vi "OE2012&OE2022_USB_Query Data.vi"(0 "VISA resource name":refnum<visa-resource-name>, 11 "Error in (no error)":errorcluster caption="error out（no error）") -> (3 "Buffer Count":u8, 4 "VISA resource  out":refnum<visa-resource-name>, 6 "Parameter Values":T1, 8 "Total Date Array":dbl[][](array[numeric]), 10 "Output String":string, 13 "Trig_Count":u8[](array[numeric]), 14 "PLL&Overload":T2, 15 "Error out":errorcluster caption="error out")   [LabVIEW 2011]
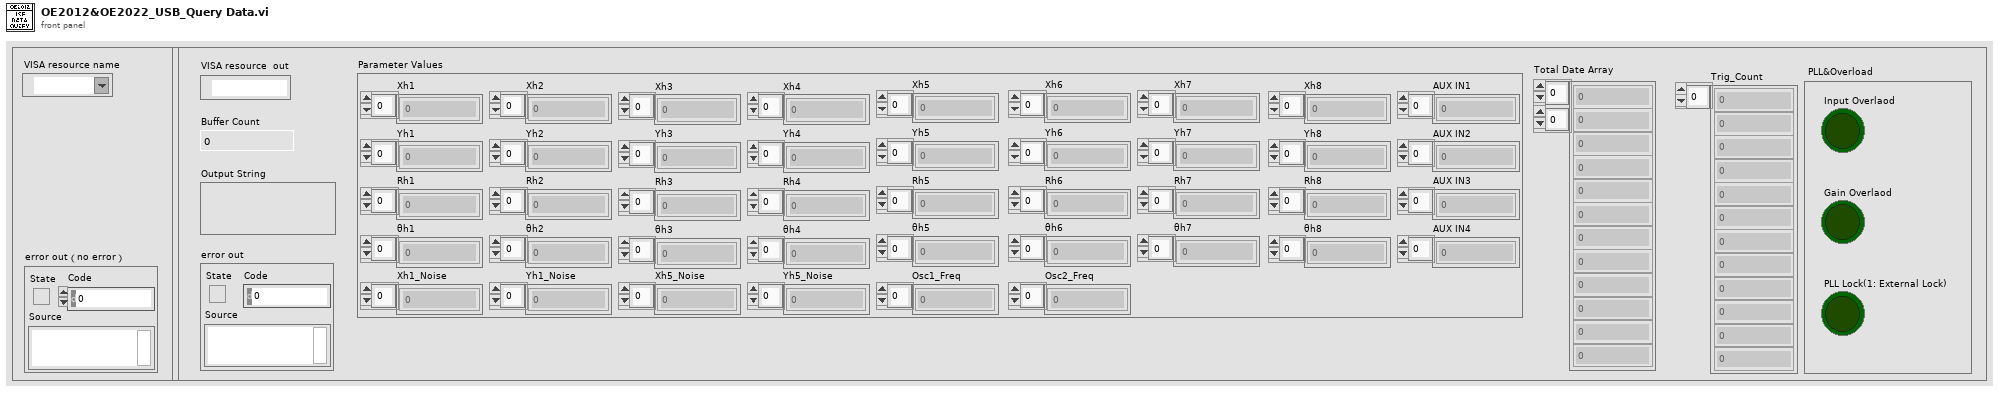
[diagram p1: front panel]
types:
  T1 = cluster{"Xh1":dbl[], "Yh1":dbl[], "Rh1":dbl[], "θh1":dbl[], "Xh1_Noise":dbl[], "Yh1_Noise":dbl[], "Xh2":dbl[], "Yh2":dbl[], "Rh2":dbl[], "θh2":dbl[], "Xh3":dbl[], "Yh3":dbl[], "Rh3":dbl[], "θh3":dbl[], "Xh4":dbl[], "Yh4":dbl[], "Rh4":dbl[], "θh4":dbl[], "Xh5":dbl[], "Yh5":dbl[], "Rh5":dbl[], "θh5":dbl[], "Xh5_Noise":dbl[], "Yh5_Noise":dbl[], "Xh6":dbl[], "Yh6":dbl[], "Rh6":dbl[], "θh6":dbl[], "Xh7":dbl[], "Yh7":dbl[], "Rh7":dbl[], "θh7":dbl[], "Xh8":dbl[], "Yh8":dbl[], "Rh8":dbl[], "θh8":dbl[], "Osc1_Freq":dbl[], "Osc2_Freq":dbl[], "AUX IN1":dbl[], "AUX IN2":dbl[], "AUX IN3":dbl[], "AUX IN4":dbl[]}
  T2 = cluster{"Input Overlaod":bool, "Gain Overlaod":bool, "PLL Lock(1: External Lock)":bool}
  T3 = cluster{"Xh1":dbl[], "Yh1":dbl[], "Rh1":dbl[], "θh1":dbl[], "Xh1_Noise":dbl[], "Yh1_Noise":dbl[], "Xh2":dbl[], "Yh2":dbl[], "Rh2":dbl[], "θh2":dbl[], "Xh3":dbl[], "Yh3":dbl[], "Rh3":dbl[], "θh3":dbl[], "Xh4":dbl[], "Yh4":dbl[], "Rh4":dbl[], "θh4":dbl[], "Xh5":dbl[], "Yh5":dbl[], "Rh5":dbl[], "θh5":dbl[], "Xh5_Noise":dbl[], "Yh5_Noise":dbl[], "Xh6":dbl[], "Yh6":dbl[], "Rh6":dbl[], "θh6":dbl[], "Xh7":dbl[], "Yh7":dbl[], "Rh7":dbl[], "θh7":dbl[], "Xh8":dbl[], "Yh8":dbl[], "Rh8":dbl[], "θh8":dbl[], "Osc1_Freq":dbl[], "Osc2_Freq":dbl[], "AUXOUT1":dbl[], "AUXOUT2":dbl[], "AUXOUT3":dbl[], "AUXOUT4":dbl[]}
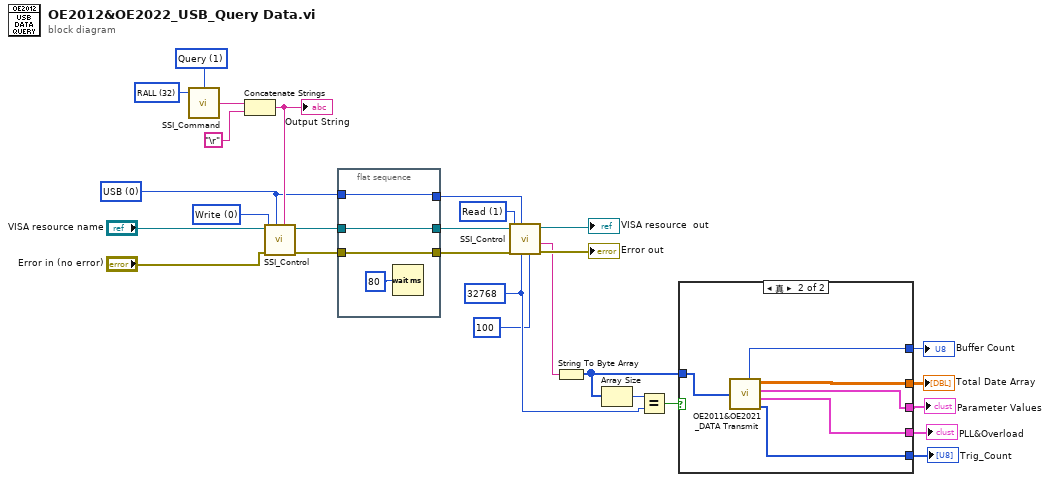
[diagram p0: block diagram]
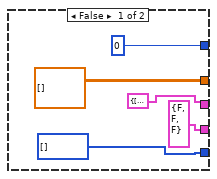
[diagram p2: hidden frame]
diagram:
  w20 = u16 0 items=["USB", "RS232", "GPIB", "Ethernet"] ("Remote Mode")
  w8 = u32 32768 ("Number of bytes")
  w14 = u16 32 items=["ISRC", "IGND", "ICPL", "ILIN", "PHAS", "FMOD", "RSLP", "FREQ", "SWPT", "SLLM", "SULM", "SSLL", "SSLG", "STLM", "SWRM", "IRNG", "SENS", "RMOD", "OFLT", "OFSL", "SYNC", "DMOD", "HARM", "DARB", "SWVT", "SLVL", "SVLL", "SVUL", "SVSL", "SVSG", "SVTM", "SVRM", "RALL", "SNAP", "OUTP", "OAUX", "COUT", "CAUX", "COFP", "CEXP", "FPOP", "OEXP", "*IDN", "*RST", "OVLD", "INOV", "GNOV", "*PLL", "SSET", "RSET", "AGAN", "APHS", "ARSV", "ASCL", "EQCD", "EQCS", "SPED", "SRAT", "SLEN", "SSLE", "STRG", "SPRM", "STRD", "PAUS", "RSET", "SPTS", "TRCA", "TEMP", "RSTU", "INHZ", "DEQU", "SADD", "ARNG", "CSPE", "ISRCD", "IGNDD", "ICPLD", "ILIND", "PHASD", "FMODD", "RSLPD", "FREQD", "SWPTD", "SLLMD", "SULMD", "SSLLD", "SSLGD", "STLMD", "SWRMD", "SENSD", "RMODD", "OFLTD", "OFSLD", "SYNCD", "HARMD", "EQCDD", "EQCSD", "SNAPD", "OUTPD", "SWVTD", "SLVLD", "SVLLD", "SVULD", "SVSLD", "SVSGD", "SVTMD", "SVRMD", "SVDCD", "ARSVD", "AGAND", "APHSD", "ASCLD", "FPOPD", "CAUXD", "OEXPD", "SPEDD", "SRATD", "SLEND", "SSLED", "STRGD", "SPRMD", "STRDD", "PAUSD", "RESTD", "SPTSD", "TRCAD", "*IDND", "*RSTD", "INOVD", "GNOVD", "*PLLD", "SSETD", "RSETD", "RALLD"] ("Command Type")
  w12 = u16 1 items=["Set", "Query"] ("Opera")
  w23 = u16 1 items=["Write", "Read"] ("Control")
  w28 = u16 0 items=["Write", "Read"] ("Control")
  n1 = call "SSI_Command.vi"("Opera"=w12, "Command Type"=w14) -> ("Output string"=w13:string)  [unwired: 2 in]
  n2 = Concatenate Strings(w13, "\r") -> (w21:string)
  "Output String" <- w21
  n3 = call "SSI_Control.vi"("Write Buffer"=w21, "Remote Mode"=w20, "Error in (no error)"="Error in (no error)", "Control"=w28, "VISA resource name"="VISA resource name") -> ("Error out"=w26:errorcluster, "VISA resource  out"=w27:refnum<visa-resource-name>)  [unwired: 3 in, 2 out]
  n4 = flat-sequence {
    tunnel: w27 -> [w32]
    tunnel: w26 -> [w31]
    tunnel: [w32] -> w25
    tunnel: [w31] -> w24
    tunnel: [w29] -> w22
    tunnel: w20 -> [w29]
    frame #0 {
      n5 = Wait (ms)(milliseconds to wait=u32 80 ("等待时间（毫秒）")) -> ()  [unwired: 1 out]
    }
  }
  n6 = call "SSI_Control.vi"("Tineout"=100, "Number of bytes"=w8, "Remote Mode"=w22, "Error in (no error)"=w24, "Control"=w23, "VISA resource name"=w25) -> ("Error out"=→"Error out":errorcluster, "Read Buffer"=w7:string, "VISA resource  out"=→"VISA resource  out":refnum<visa-resource-name>)  [unwired: 2 in, 1 out]
  n7 = String To Byte Array(string=w7) -> (unsigned byte array=w9:u8[])
  n8 = Array Size(array=w9) -> (size(s)=w10:i32)
  n9 = Equal?(x=w10, y=w8) -> (x = y?=w11:bool)
  n10 = case shown="真" w11 {
    tunnel: [u8 0 w38] -> w6
    tunnel: w9 -> [_ w43]
    tunnel: [dbl[][] [] ("Total Data Array") w42] -> w5
    tunnel: [T2 {"Input Overlaod"=FALSE, "Gain Overlaod"=FALSE, "PLL Lock(1: External Lock)"=FALSE} ("PLL&Overload") w41] -> w4
    tunnel: [i32[] [] w40] -> w3
    tunnel: [T3 {"Xh1"=[], "Yh1"=[], "Rh1"=[], "θh1"=[], "Xh1_Noise"=[], "Yh1_Noise"=[], "Xh2"=[], "Yh2"=[], "Rh2"=[], "θh2"=[], "Xh3"=[], "Yh3"=[], "Rh3"=[], "θh3"=[], "Xh4"=[], "Yh4"=[], "Rh4"=[], "θh4"=[], "Xh5"=[], "Yh5"=[], "Rh5"=[], "θh5"=[], "Xh5_Noise"=[], "Yh5_Noise"=[], "Xh6"=[], "Yh6"=[], "Rh6"=[], "θh6"=[], "Xh7"=[], "Yh7"=[], "Rh7"=[], "θh7"=[], "Xh8"=[], "Yh8"=[], "Rh8"=[], "θh8"=[], "Osc1_Freq"=[], "Osc2_Freq"=[], "AUXOUT1"=[], "AUXOUT2"=[], "AUXOUT3"=[], "AUXOUT4"=[]} ("Parameter Values") w39] -> w2
    frame False {
    }
    frame True {
      n11 = call "OE2011&OE2021_DATA Transmit.vi"("Input Data"=w43) -> ("Trig_Count"=w40:u8[], "PLL&Overload"=w41:T2, "Parameter Values"=w39:T1, "Total Date Array"=w42:dbl[][], "Buffer Count"=w38:u8)
    }
  }
  "Buffer Count" <- w6
  "Trig_Count" <- w3
  "PLL&Overload" <- w4
  "Total Date Array" <- w5
  "Parameter Values" <- w2
